vi "Initialize.vi"(8 "error in (no error)":errorcluster, 10 "Top Level Diagram":refnum<vi>, 11 "DMA Loop in":refnum<class "DMA Loop.lvclass">) -> (0 "error out":errorcluster, 3 "DMA Loop out":refnum<class "DMA Loop.lvclass">)   [LabVIEW 2015, in "DMA Loop.lvclass"]
uses:
  DMA Loop.lvclass
  <vilib>/Utility/miscctls.llb/LVPointTypeDef.ctl
  Structures/Structures.lvclass/Structures.ctl
  Loop/Loop.lvclass/Loop.ctl
  Structures/Write Structure.vi
  Loop/Write Loop Structure.vi
  Structures/Write Location.vi
  Structures/Write Diagram.vi
  Structures/Structures.lvclass
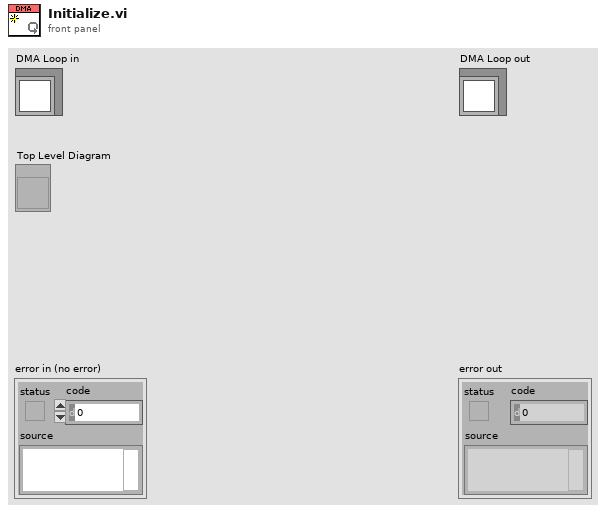
[diagram p1: front panel]
types:
  T1 = typedef "LVPointTypeDef.ctl" = cluster{"Horizontal":i16, "Vertical":i16}
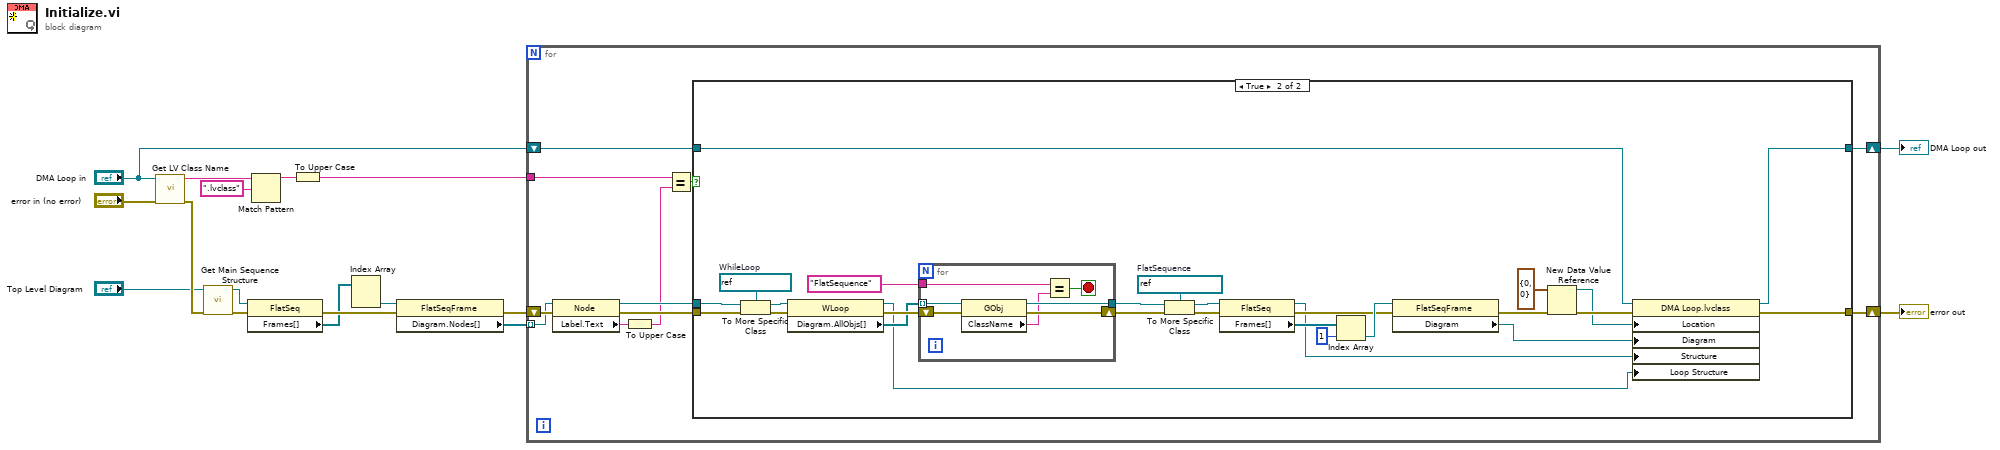
[diagram p0: block diagram]
diagram:
  n1 = call <vilib>:"Get LV Class Name.vi"("error in (no error)"="error in (no error)", "object"="DMA Loop in") -> ("error out"=w8:errorcluster, "class name"=w12:string)  [unwired: 8 in]
  n2 = call "Get Main Sequence Structure.vi"("error in (no error)"=w8, "Top Level Diagram"="Top Level Diagram") -> ("error out"=w7:errorcluster, "Main.SeqStructure"=w6:refnum<vi>)  [unwired: 8 in]
  n3 = property class="FlatSeq"(reference=w6, error in=w7) -> (error out=w14:errorcluster, "Frames[]"=w13:refnum<vi>[])  [unwired: 1 out]
  n4 = Match Pattern(string=w12, regular expression=".lvclass") -> (before substring=w10:string)  [unwired: 1 in, 3 out]
  n5 = To Upper Case(1:w10) -> (0:w9:string)
  n6 = Index Array(array=w13) -> (element #2=w17:refnum<vi>)  [unwired: 2 in, 1 out]
  n7 = property class="FlatSeqFrame"(reference=w17, error in=w14) -> (error out=w16:errorcluster, "Diagram.Nodes[]"=w15:refnum<vi>[])  [unwired: 1 out]
  n8 = for {
    tunnel: w15 -> [w27] mode=indexing
    shift-right: [w23] -> w5
    shift-left: w16 -> [w28]
    tunnel: w9 -> [w21]
    shift-right: [w19] -> w1
    shift-left: "DMA Loop in" -> [w20]
    n9 = property class="Node"(reference=w27, error in=w28) -> (reference out=w25:refnum<vi>, error out=w24:errorcluster, "Label.Text"=w26:string)
    n10 = To Upper Case(1:w26) -> (0:w22:string)
    n11 = Equal?(x=w21, y=w22) -> (x = y?=w18:bool)
    n12 = case shown="True" w18 {
      tunnel: w25 -> [_ w56]
      tunnel: w24 -> [w30 w57]
      tunnel: [w30 w41] -> w23
      tunnel: w20 -> [w29 w38]
      tunnel: [w29 w40] -> w19
      frame False {
      }
      frame True {
        w55 = refnum<vi> refnum  # WhileLoop
        w50 = refnum<vi> refnum  # FlatSequence
        n13 = To More Specific Class(target class=w55, reference=w56, error in=w57) -> (specific class reference=w37:refnum<vi>, error out=w54:errorcluster)
        n14 = property class="WLoop"(reference=w37, error in=w54) -> (reference out=w36:refnum<vi>, error out=w53:errorcluster, "Diagram.AllObjs[]"=w52:refnum<vi>[])
        n15 = for {
          shift-right: [w63] -> w51
          shift-left: w53 -> [w64]
          tunnel: w52 -> [w62] mode=indexing
          tunnel: "FlatSequence" ("name/order") -> [w61]
          tunnel: [w59] -> w48
          stop <- w60 stop-if-true
          n16 = property class="GObj"(reference=w62, error in=w64) -> (reference out=w59:refnum<vi>, error out=w63:errorcluster, "ClassName"=w58:string)
          n17 = Equal?(x=w61, y=w58) -> (x = y?=w60:bool)
        }
        n18 = To More Specific Class(target class=w50, reference=w48, error in=w51) -> (specific class reference=w47:refnum<vi>, error out=w46:errorcluster)
        n19 = property class="FlatSeq"(reference=w47, error in=w46) -> (reference out=w39:refnum<vi>, error out=w43:errorcluster, "Frames[]"=w42:refnum<vi>[])
        n20 = Index Array(array=w42, index=1) -> (element=w44:refnum<vi>)
        n21 = property class="FlatSeqFrame"(reference=w44, error in=w43) -> (error out=w33:errorcluster, "Diagram"=w35:refnum<vi>)  [unwired: 1 out]
        n22 = New Data Value Reference(data value=T1 {"Horizontal"=0, "Vertical"=0} ("location out"), error in=w33) -> (data value reference=w31:refnum<data-value>, error out=w32:errorcluster)
        n23 = property class="DMA Loop.lvclass"(reference=w38, error in=w32, "Location"=w31, "Diagram"=w35, "Structure"=w39, "Loop Structure"=w36) -> (reference out=w40:refnum<class "DMA Loop.lvclass">, error out=w41:errorcluster)
      }
    }
  }
  "error out" <- w5
  "DMA Loop out" <- w1
